vi "Get On State on Multiple Controls.vi"(11 "Controls":refnum<vi>[](array[refnum]) caption="컨트롤") -> (3 "results":bool[](array[boolean]))   [LabVIEW 2018, in "Library-Ctrl.lvlib"]
uses:
  Library-Ctrl.lvlib
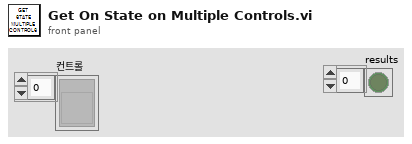
[diagram p1: front panel]
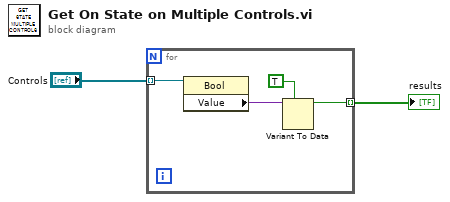
[diagram p0: block diagram]
diagram:
  n1 = for {
    tunnel: "Controls" -> [w6] mode=indexing
    tunnel: [w3] -> w1 mode=indexing
    n2 = property class="Bool"(reference=w6) -> ("Value"=w5:variant)  [unwired: 1 in, 2 out]
    n3 = Variant To Data(type=TRUE, Variant=w5) -> (data=w3:bool)  [unwired: 1 in, 1 out]
  }
  "results" <- w1
